vi "clearStoredSession.vi"(8 "error in":errorcluster, 10 "Client ID":string, 11 "MQTT Server":refnum<class "Server.lvclass">) -> (0 "error out":errorcluster, 1 "Session Cleared":bool, 2 "Client ID dup":string, 3 "MQTT Server out":refnum<class "Server.lvclass">)   [LabVIEW 2013, in "MQTT Server.lvlib" / "Server.lvclass"]
uses:
  Server.lvclass
  StoredSessions/StoredSessions.lvclass
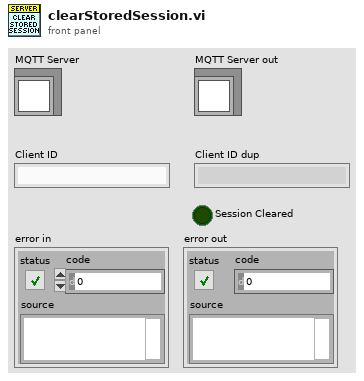
[diagram p1: front panel]
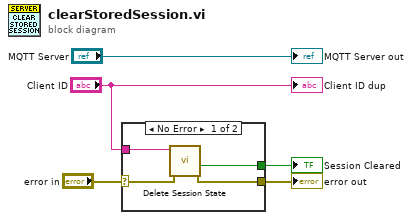
[diagram p0: block diagram]
diagram:
  n1 = case shown="No Error" "error in" {
    selector: "error in" -> [w7 w10]
    tunnel: [w6 w10] -> w4
    tunnel: "Client ID" -> [w9 _]
    tunnel: [w8 _] -> w3
    frame No Error {
      n2 = call "Delete Session State.vi"("error in (no error)"=w7, "Client ID"=w9) -> ("error out"=w6:errorcluster, "Found?"=w8:bool)  [unwired: 8 in]
    }
    frame Error {
    }
  }
  "error out" <- w4
  "Session Cleared" <- w3
  "Client ID dup" <- "Client ID"
  "MQTT Server out" <- "MQTT Server"
